vi "getAll.vi"(8 "error in (no error)":errorcluster, 11 "instrument.PPMS2 in":refnum<class "instrument.PPMS2.lvclass">) -> (0 "error out":errorcluster, 2 "getAll":variant, 3 "instrument.PPMS2 out":refnum<class "instrument.PPMS2.lvclass">)   [LabVIEW 2016, in "instrument.PPMS2.lvclass"]
uses:
  instrument.PPMS2.lvclass
  Typedefs/getAll--PPMS2--cluster.ctl
  Typedefs/Temperature Status--PPMS2--ring.ctl
  Typedefs/Magnet Status--PPMS2--ring.ctl
  instrument.PPMS2.lvclass/instrument.PPMS2.ctl
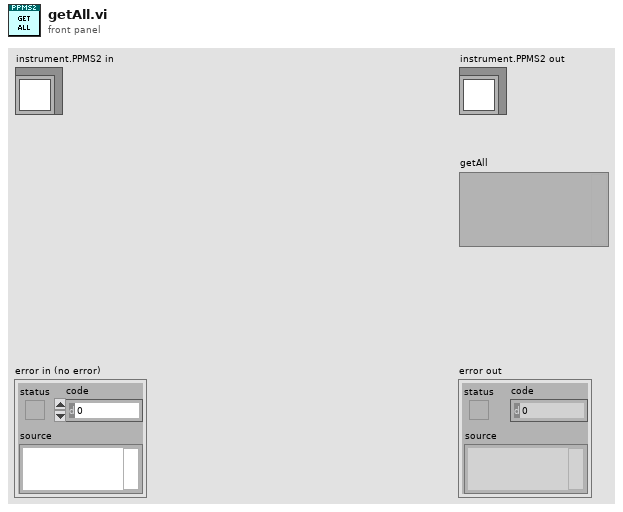
[diagram p1: front panel]
types:
  T1 = typedef "instrument.PPMS2.lvclass/getAll--PPMS2--cluster.ctl" = cluster{"PPMS 2 Helium Level":dbl, "PPMS 2 Temperature":dbl, "PPMS 2 Temperature Status":T2, "PPMS 2 Magnetic Field":dbl, "PPMS 2 Magnet Status":T3, "PPMS 2 Position":dbl}
  T2 = typedef "instrument.PPMS2.lvclass/Temperature Status--PPMS2--ring.ctl" = i32
  T3 = typedef "instrument.PPMS2.lvclass/Magnet Status--PPMS2--ring.ctl" = i32
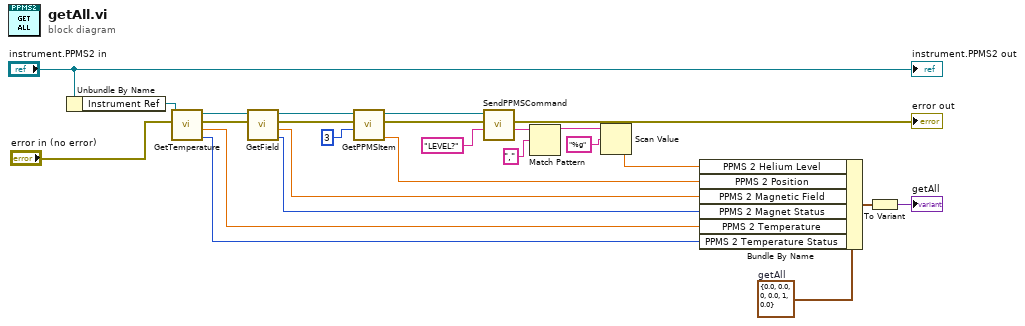
[diagram p0: block diagram]
diagram:
  w14 = T1 {"PPMS 2 Helium Level"=0.0, "PPMS 2 Temperature"=0.0, "PPMS 2 Temperature Status"=0, "PPMS 2 Magnetic Field"=0.0, "PPMS 2 Magnet Status"=1, "PPMS 2 Position"=0.0}  # getAll
  n1 = Unbundle By Name("instrument.PPMS2 in") -> ("Instrument Ref"=w8:refnum<k24>)
  n2 = call "GetTemperature.vi"("error in (no error)"="error in (no error)", "Instrument Ref In"=w8) -> ("Temperature\nStatus"=w3:i32, "Temperature"=w12:dbl, "error out"=w24:errorcluster, "Instrument Ref Out"=w23:refnum<k24>)  [unwired: 3 in, 1 out]
  n3 = call "GetField.vi"("error in (no error)"=w24, "Instrument Ref In"=w23) -> ("Field\nStatus"=w4:i32, "Field"=w13:dbl, "error out"=w20:errorcluster, "Instrument Ref Out"=w21:refnum<k24>)  [unwired: 3 in, 1 out]
  n4 = call "GetPPMSItem.vi"("Channel"=3, "error in (no error)"=w20, "Instrument Ref In"=w21) -> ("Result"=w1:dbl, "error out"=w16:errorcluster, "Instrument Ref Out"=w17:refnum<k24>)  [unwired: 1 in, 1 out]
  n5 = call "SendPPMSCommand.vi"("PpmsCommand"="LEVEL?", "error in (no error)"=w16, "Instrument Ref In"=w17) -> ("PpmsReply"=w25:string, "error out"=→"error out":errorcluster)  [unwired: 4 in, 3 out]
  n6 = Match Pattern(string=w25, regular expression=",") -> (before substring=w11:string)  [unwired: 1 in, 3 out]
  n7 = Scan Value(string=w11, format string="%g") -> (value=w2:dbl)  [unwired: 1 in, 1 out]
  n8 = Bundle By Name(cluster=w14, "PPMS 2 Helium Level"=w2, "PPMS 2 Position"=w1, "PPMS 2 Magnetic Field"=w13, "PPMS 2 Magnet Status"=w4, "PPMS 2 Temperature"=w12, "PPMS 2 Temperature Status"=w3) -> (w5:T1)
  n9 = To Variant(anything=w5) -> (Variant=→"getAll":variant)
  "instrument.PPMS2 out" <- "instrument.PPMS2 in"
